vi "Generic PAS Operation.vi"   [LabVIEW 2012]
uses:
  Reusable/Instrument/Instrument.lvclass
  Reusable/Instrument/state.ctl
  Reusable/PAS/Main/PAS.lvclass
types:
  T1 = typedef "Instrument.lvclass/state.ctl" = enum8{"Configure", "Acquire", "Wait", "Quit", "Handle Error", "NOOP"}
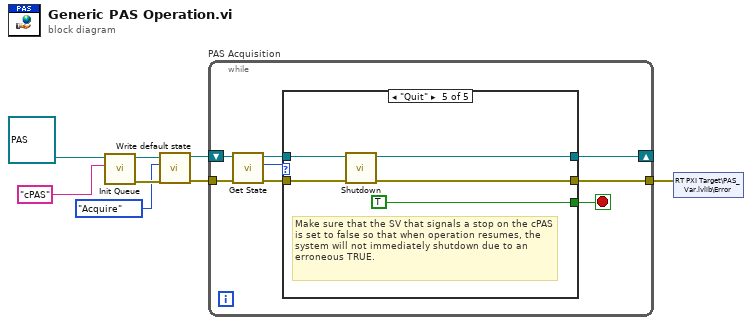
[diagram p0: block diagram]
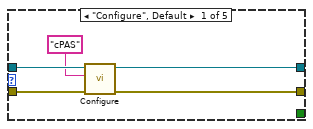
[diagram p2: hidden frame]
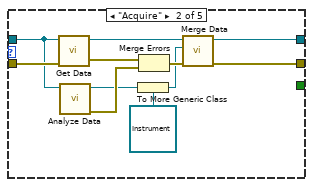
[diagram p3: hidden frame]
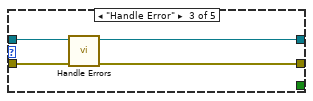
[diagram p4: hidden frame]
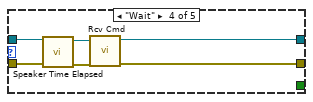
[diagram p5: hidden frame]
diagram:
  n1 = call "Init Queue.vi"("queue_name"="cPAS", "Instrument in"=refnum<class "PAS.lvclass"> refnum ("PASIn")) -> ("error out"=w7:errorcluster, "Instrument out"=w8:refnum<class "PAS.lvclass">)  [unwired: 8 in]
  n2 = call "Write default state.vi"("error in (no error)"=w7, "instr state"=state."Acquire", "Instrument in"=w8) -> ("error out"=w6:errorcluster, "Instrument out"=w2:refnum<class "PAS.lvclass">)  [unwired: 7 in]
  n3 = while "PAS Acquisition" {
    tunnel: w6 -> [w16]
    shift-right: [w9] -> _
    shift-left: w2 -> [w15]
    tunnel: [w13] -> w1
    stop <- w12 stop-if-true
    n4 = call "Get State.vi"("error in"=w16, "Instrument in"=w15) -> ("error out"=w14:errorcluster, "default state"=w11:T1, "Instrument out"=w10:refnum<class "PAS.lvclass">)  [unwired: 7 in]
    n5 = case shown="\"Quit\"" w11 {
      tunnel: w10 -> [w21 w31 w36 w40 w46]
      tunnel: w14 -> [w20 w32 w35 w39 w45]
      tunnel: [_ _ _ _ TRUE] -> w12
      tunnel: [w19 w23 w34 w42 w44] -> w9
      tunnel: [w18 w22 w33 w41 w43] -> w13
      frame "Configure", Default {
        n6 = call-dynamic "Configure.vi"("error in"=w20, "name"="cPAS", "PAS in"=w21) -> ("error out"=w18:errorcluster, "PAS out"=w19:refnum<class "PAS.lvclass">)  [unwired: 7 in]
      }
      frame "Acquire" {
        n7 = call-dynamic "Get Data.vi"("error in"=w32, "PAS in"=w31) -> ("error out"=w30:errorcluster, "PAS out"=w29:refnum<class "PAS.lvclass">)  [unwired: 8 in]
        n8 = call-dynamic "Analyze Data.vi"("PAS in"=w31) -> ("error out"=w27:errorcluster, "PAS out"=w26:refnum<class "PAS.lvclass">)  [unwired: 9 in]
        n9 = To More Generic Class(target class=refnum<class "Instrument.lvclass"> refnum ("Instrument.lvclass"), reference=w26) -> (generic class reference=w25:refnum<class "Instrument.lvclass">)
        n10 = Merge Errors(w30, w27) -> (w28:errorcluster)
        n11 = call-dynamic "Merge Data.vi"("error in"=w28, "Analyzed"=w25, "Acquired"=w29) -> ("error out"=w22:errorcluster, "PAS out"=w23:refnum<class "PAS.lvclass">)  [unwired: 7 in]
      }
      frame "Handle Error" {
        n12 = call-dynamic "Handle Errors.vi"("error in"=w35, "PAS in"=w36) -> ("error out"=w33:errorcluster, "PAS out"=w34:refnum<class "PAS.lvclass">)  [unwired: 7 in, 1 out]
      }
      frame "Wait" {
        n13 = call-dynamic "Speaker Time Elapsed.vi"("error in"=w39, "PAS in"=w40) -> ("error out"=w37:errorcluster, "PAS out"=w38:refnum<class "PAS.lvclass">)  [unwired: 7 in, 1 out]
        n14 = call-dynamic "Rcv Cmd.vi"("error in"=w37, "PAS in"=w38) -> ("error out"=w41:errorcluster, "PAS out"=w42:refnum<class "PAS.lvclass">)  [unwired: 8 in]
      }
      frame "Quit" {
        # "Make sure that the SV that signals a stop on the cPAS is set to false so that when operation resumes, the system will not immediately shutdown due to an erroneous TRUE."
        n15 = call-dynamic "Shutdown.vi"("error in"=w45, "PAS in"=w46) -> ("error out"=w43:errorcluster, "PAS out"=w44:refnum<class "PAS.lvclass">)  [unwired: 8 in]
      }
    }
  }
  n16 = shared-variable "RT PXI Target\\PAS_Var.lvlib\\Error"(w1) -> ()  [unwired: 1 in, 1 out]
